vi "AddArrow.vi"(10 "Slide":dbl, 11 "Refnum in":T1) -> (3 "Refnum out":T1)   [LabVIEW 2018]
uses:
  <vilib>/vision/Image Controls.llb/IMAQ Image.ctl
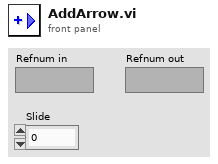
[diagram p1: front panel]
types:
  T1 = typedef "IMAQ Image.ctl" = refnum<image>
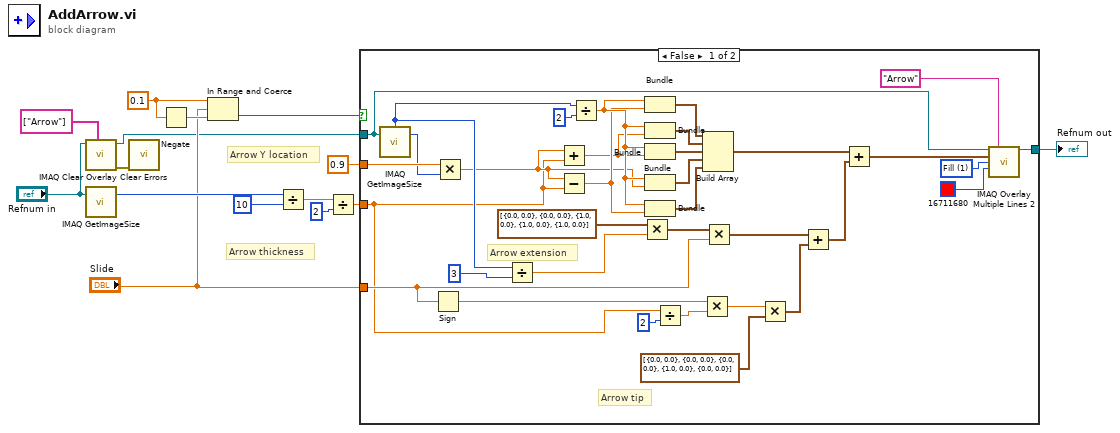
[diagram p0: block diagram]
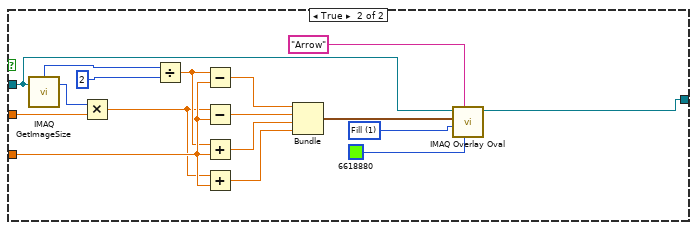
[diagram p2: hidden frame]
diagram:
  w6 = 0.1 ("upper limit")
  # "Arrow Y location"
  # "Arrow thickness"
  n1 = call "IMAQ Clear Overlay"("Groups"=string[] ["Arrow"], "Image"="Refnum in") -> ("error out"=w3:errorcluster, "Image Out"=w2:T1)  [unwired: 8 in]
  n2 = call "IMAQ GetImageSize"("Image"="Refnum in") -> ("Y Resolution"=w14:i32)  [unwired: 3 in, 2 out]
  n3 = call <vilib>:"Clear Errors.vi"("error in (no error)"=w3) -> ()  [unwired: 5 in, 2 out]
  n4 = Negate(x=w6) -> (-x=w7:dbl)
  n5 = In Range and Coerce(upper limit=w6, x="Slide", lower limit=w7) -> (In Range?=w4:bool)  [unwired: 1 out]
  n6 = Divide(x=w14, y=10) -> (x/y=w11:dbl)
  n7 = Divide(x=w11, y=2) -> (x/y=w9:dbl)
  n8 = case shown="False" w4 {
    tunnel: [w49 w66] -> w1
    tunnel: w2 -> [w34 w63]
    tunnel: "Slide" -> [w38 _]
    tunnel: w9 -> [w18 w59]
    tunnel: 0.9 -> [w31 w51]
    frame False {
      w48 = u32 1 items=["Frame", "Fill"] ("Drawing Mode (Frame)")
      # "Arrow tip"
      # "Arrow extension"
      n9 = call "IMAQ GetImageSize"("Image"=w34) -> ("Y Resolution"=w30:i32, "X Resolution"=w23:i32)  [unwired: 3 in, 1 out]
      n10 = Sign(1:w38) -> (0:w41:dbl)
      n11 = Multiply(x=w31, y=w30) -> (x*y=w19:dbl)
      n12 = Divide(x=w23, y=3) -> (x/y=w33:dbl)
      n13 = Add(x=w19, y=w18) -> (x+y=w17:dbl)
      n14 = Subtract(x=w19, y=w18) -> (x-y=w20:dbl)
      n15 = Divide(x=w23, y=2) -> (x/y=w21:dbl)
      n16 = Multiply(x=cluster{"X":dbl, "Y":dbl}[] [{"X"=0.0, "Y"=0.0}, {"X"=0.0, "Y"=0.0}, {"X"=1.0, "Y"=0.0}, {"X"=1.0, "Y"=0.0}, {"X"=1.0, "Y"=0.0}] ("Line End Points"), y=w33) -> (x*y=w43:cluster{"X":dbl, "Y":dbl}[])
      n17 = Bundle(w21, w20) -> (w25:cluster{dbl, dbl})  [unwired: 1 in]
      n18 = Bundle(w21, w17) -> (w26:cluster{dbl, dbl})  [unwired: 1 in]
      n19 = Bundle(w21, w17) -> (w27:cluster{dbl, dbl})  [unwired: 1 in]
      n20 = Bundle(w21, w19) -> (w28:cluster{dbl, dbl})  [unwired: 1 in]
      n21 = Bundle(w21, w20) -> (w29:cluster{dbl, dbl})  [unwired: 1 in]
      n22 = Divide(x=w18, y=2) -> (x/y=w36:dbl)
      n23 = Multiply(x=w41, y=w36) -> (x*y=w37:dbl)
      n24 = Build Array(w25, w26, w27, w28, w29) -> (w24:cluster{dbl, dbl}[])
      n25 = Multiply(x=w43, y=w38) -> (x*y=w44:cluster{"X":dbl, "Y":dbl}[])
      n26 = Multiply(x=w37, y=cluster{"X":dbl, "Y":dbl}[] [{"X"=0.0, "Y"=0.0}, {"X"=0.0, "Y"=0.0}, {"X"=0.0, "Y"=0.0}, {"X"=1.0, "Y"=0.0}, {"X"=0.0, "Y"=0.0}] ("Line End Points")) -> (x*y=w39:cluster{"X":dbl, "Y":dbl}[])
      n27 = Add(x=w44, y=w39) -> (x+y=w40:cluster{"X":dbl, "Y":dbl}[])
      n28 = Add(x=w24, y=w40) -> (x+y=w45:cluster{dbl, dbl}[])
      n29 = call "IMAQ Overlay Multiple Lines 2"("Image"=w34, "Group"="Arrow", "Line End Points"=w45, "Drawing Mode (Frame)"=w48, "Color"=u32 16711680) -> ("Image Out"=w49:T1)  [unwired: 9 in, 1 out]
    }
    frame True {
      w64 = u32 1 items=["Frame", "Fill"] ("Drawing Mode (Frame)")
      n30 = call "IMAQ GetImageSize"("Image"=w63) -> ("Y Resolution"=w53:i32, "X Resolution"=w61:i32)  [unwired: 3 in, 1 out]
      n31 = Multiply(x=w53, y=w51) -> (x*y=w52:dbl)
      n32 = Divide(x=w61, y=2) -> (x/y=w57:dbl)
      n33 = Subtract(x=w57, y=w59) -> (x-y=w58:dbl)
      n34 = Subtract(x=w52, y=w59) -> (x-y=w54:dbl)
      n35 = Add(x=w57, y=w59) -> (x+y=w56:dbl)
      n36 = Add(x=w52, y=w59) -> (x+y=w55:dbl)
      n37 = Bundle(w58, w54, w56, w55) -> (w62:cluster{dbl, dbl, dbl, dbl})  [unwired: 1 in]
      n38 = call "IMAQ Overlay Oval"("Color"=u32 6618880, "Group"="Arrow", "Drawing Mode (Frame)"=w64, "Bounding Rectangle"=w62, "Image"=w63) -> ("Image Out"=w66:T1)  [unwired: 5 in, 1 out]
    }
  }
  "Refnum out" <- w1
